vi "Parse Vector Line.vi"(11 "string":string) -> (1 "perform test":bool, 3 "string out":string)   [LabVIEW 2017]
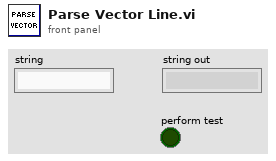
[diagram p1: front panel]
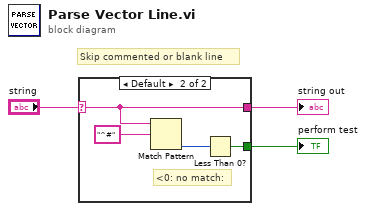
[diagram p0: block diagram]
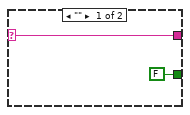
[diagram p2: hidden frame]
diagram:
  # "Skip commented or blank line"
  n1 = case shown="Default" "string" {
    selector: "string" -> [w5 w6]
    tunnel: [FALSE w7] -> w1
    tunnel: [w5 w6] -> w2
    frame "" {
    }
    frame Default {
      # "<0: no match:"
      n2 = Match Pattern(string=w6, regular expression="^#") -> (offset past match=w8:i32)  [unwired: 1 in, 3 out]
      n3 = Less Than 0?(x=w8) -> (x < 0?=w7:bool)
    }
  }
  "perform test" <- w1
  "string out" <- w2
